vi "addImageToQueue.vi"(8 "error in (no error)":errorcluster, 10 "ImageData":T1, 11 "Camera in":refnum<class "Camera.lvclass">) -> (0 "error out":errorcluster, 3 "Camera out":refnum<class "Camera.lvclass">)   [LabVIEW 2009, in "Hardware.lvlib" / "Channels.lvlib" / "Camera.lvclass"]
uses:
  Camera.lvclass
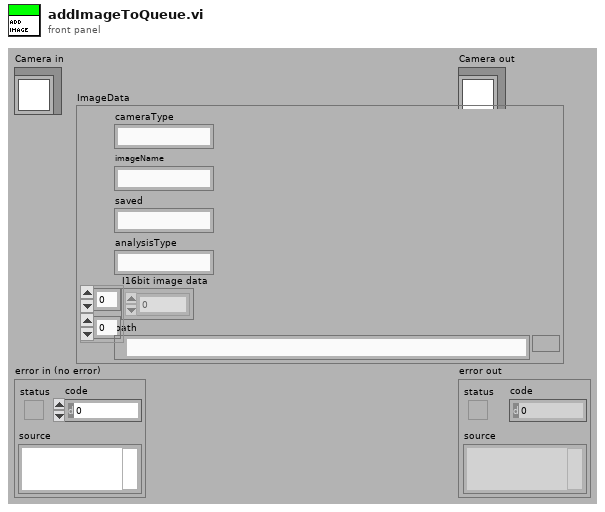
[diagram p1: front panel]
types:
  T1 = cluster{"cameraType":string, "imageName":string, "saved":string, "analysisType":string, "I16bit image data":u16[][], "path":path}
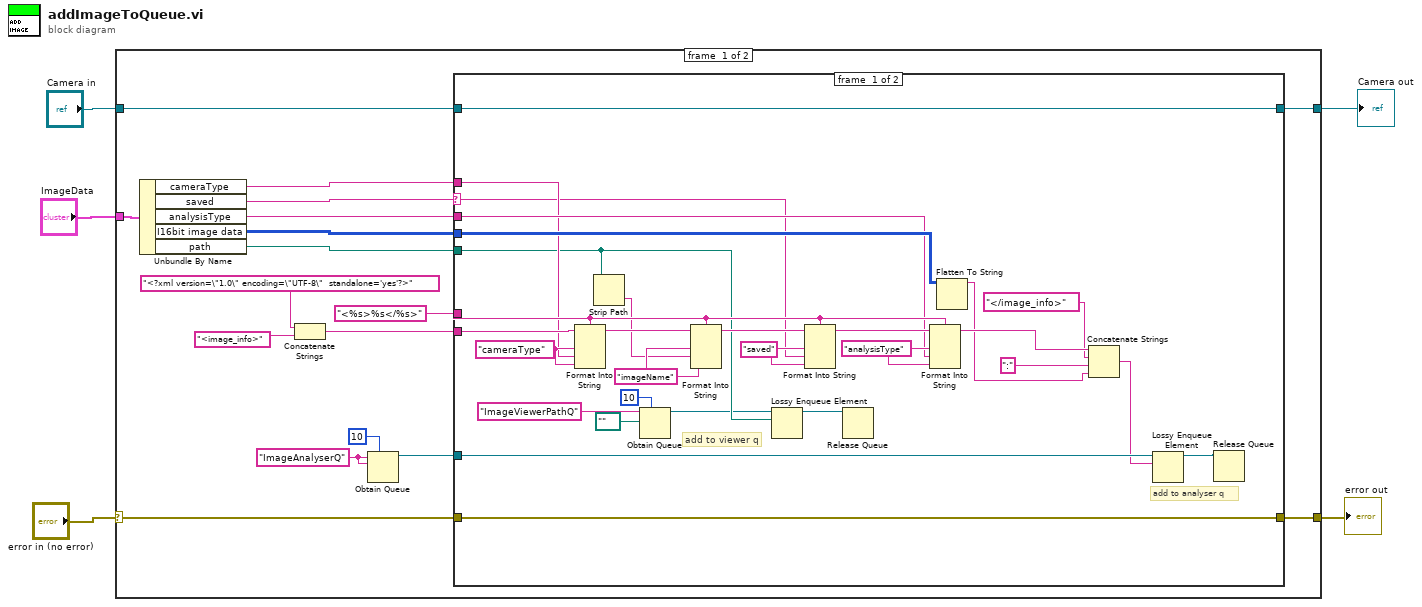
[diagram p0: block diagram]
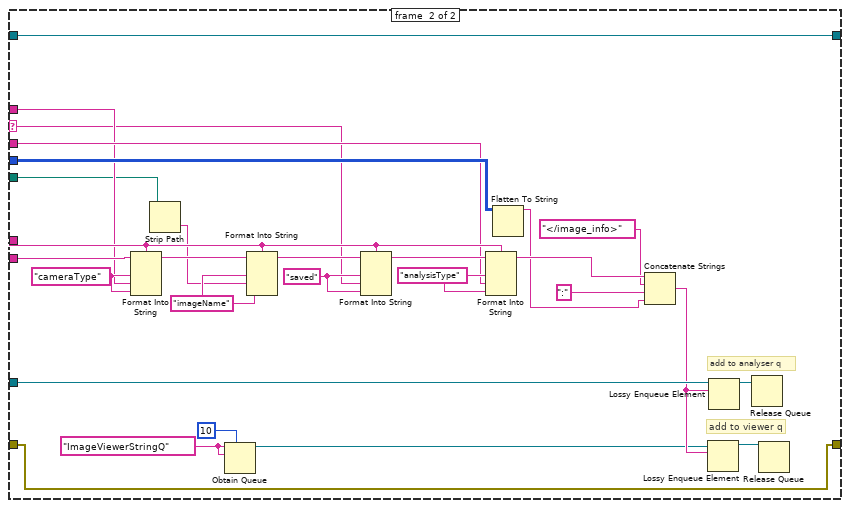
[diagram p2: hidden frame]
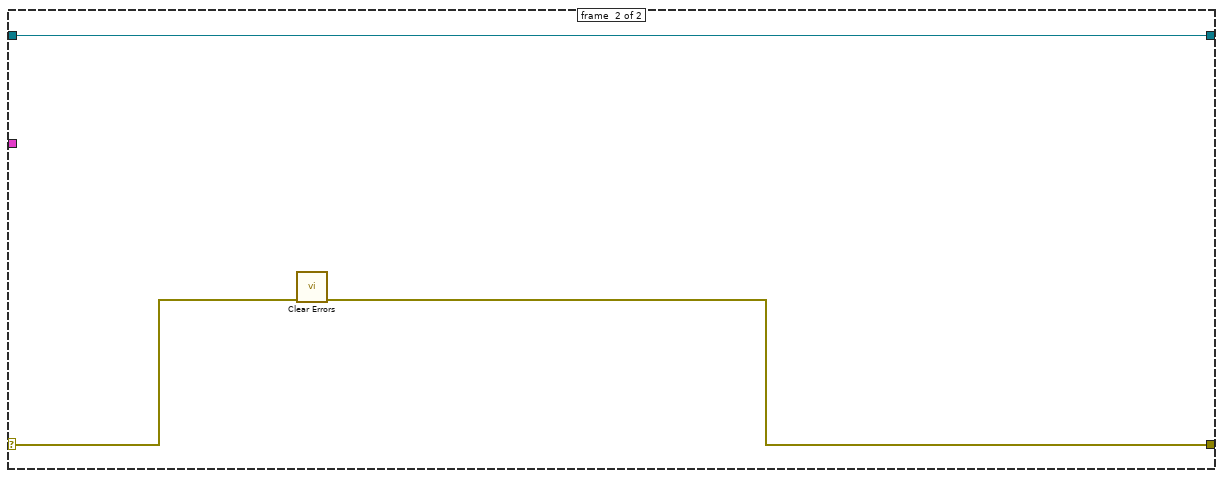
[diagram p3: hidden frame]
diagram:
  n1 = case shown="No Error" "error in (no error)" {
    selector: "error in (no error)" -> [w7 w82]
    tunnel: [w6 w80] -> w4
    tunnel: [w19 w81] -> w2
    tunnel: "Camera in" -> [w21 w81]
    tunnel: "ImageData" -> [w22 _]
    frame #0 {
      w10 = "ImageAnalyserQ"
      n2 = Unbundle By Name(w22) -> ("cameraType"=w18:string, "saved"=w20:string, "analysisType"=w17:string, "I16bit image data"=w16:u16[][], "path"=w15:path)
      n3 = Concatenate Strings("<?xml version=\"1.0\" encoding=\"UTF-8\"  standalone='yes'?>", "<image_info>") -> (w12:string)
      n4 = Obtain Queue(max queue size (-1, unlimited)=10, name (unnamed)=w10, element data type=w10) -> (queue out=w8:refnum<queue>)  [unwired: 2 in, 2 out]
      n5 = case shown="\"true\"" w20 {
        selector: w20 -> [w33 w61]
        tunnel: w21 -> [w51 w79]
        tunnel: [w51 w79] -> w19
        tunnel: w18 -> [w34 w62]
        tunnel: w17 -> [w35 w63]
        tunnel: w16 -> [w37 w65]
        tunnel: w15 -> [w32 w60]
        tunnel: w12 -> [w40 w68]
        tunnel: "<%s>%s</%s>" -> [w39 w67]
        tunnel: w8 -> [w31 w59]
        tunnel: w7 -> [w23 w52]
        tunnel: [w23 w52] -> w6
        frame #0 {
          w48 = "analysisType"
          w46 = "saved"
          w42 = "imageName" ("Key")
          w41 = "cameraType"
          # "add to analyser q"
          # "add to viewer q"
          n6 = Format Into String(format string=w39, initial string=w40, w41, w34, w41) -> (resulting string=w44:string)  [unwired: 1 in, 1 out]
          n7 = Strip Path(path=w32) -> (name=w38:string)  [unwired: 1 out]
          n8 = Obtain Queue(max queue size (-1, unlimited)=10, name (unnamed)="ImageViewerPathQ", element data type=path "") -> (queue out=w26:refnum<queue>)  [unwired: 2 in, 2 out]
          n9 = Format Into String(format string=w39, initial string=w44, w42, w38, w42) -> (resulting string=w45:string)  [unwired: 1 in, 1 out]
          n10 = Lossy Enqueue Element(queue=w26, element=w32) -> (queue out=w25:refnum<queue>)  [unwired: 1 in, 3 out]
          n11 = Format Into String(format string=w39, initial string=w45, w46, w33, w46) -> (resulting string=w49:string)  [unwired: 1 in, 1 out]
          n12 = Release Queue(queue=w25) -> ()  [unwired: 2 in, 3 out]
          n13 = Format Into String(format string=w39, initial string=w49, w48, w35, w48) -> (resulting string=w50:string)  [unwired: 1 in, 1 out]
          n14 = Flatten To String(anything=w37) -> (data string=w36:string)  [unwired: 3 in, 2 out]
          n15 = Concatenate Strings(w50, "</image_info>", ":", w36) -> (w30:string)
          n16 = Lossy Enqueue Element(queue=w31, element=w30) -> (queue out=w24:refnum<queue>)  [unwired: 1 in, 3 out]
          n17 = Release Queue(queue=w24) -> ()  [unwired: 2 in, 3 out]
        }
        frame #1 {
          w56 = "ImageViewerStringQ"
          w76 = "analysisType"
          w74 = "saved"
          w70 = "imageName" ("Key")
          w69 = "cameraType"
          # "add to analyser q"
          # "add to viewer q"
          n18 = Format Into String(format string=w67, initial string=w68, w69, w62, w69) -> (resulting string=w72:string)  [unwired: 1 in, 1 out]
          n19 = Strip Path(path=w60) -> (name=w66:string)  [unwired: 1 out]
          n20 = Obtain Queue(max queue size (-1, unlimited)=10, name (unnamed)=w56, element data type=w56) -> (queue out=w55:refnum<queue>)  [unwired: 2 in, 2 out]
          n21 = Format Into String(format string=w67, initial string=w72, w70, w66, w70) -> (resulting string=w73:string)  [unwired: 1 in, 1 out]
          n22 = Format Into String(format string=w67, initial string=w73, w74, w61, w74) -> (resulting string=w77:string)  [unwired: 1 in, 1 out]
          n23 = Format Into String(format string=w67, initial string=w77, w76, w63, w76) -> (resulting string=w78:string)  [unwired: 1 in, 1 out]
          n24 = Flatten To String(anything=w65) -> (data string=w64:string)  [unwired: 3 in, 2 out]
          n25 = Concatenate Strings(w78, "</image_info>", ":", w64) -> (w58:string)
          n26 = Lossy Enqueue Element(queue=w55, element=w58) -> (queue out=w53:refnum<queue>)  [unwired: 1 in, 3 out]
          n27 = Lossy Enqueue Element(queue=w59, element=w58) -> (queue out=w54:refnum<queue>)  [unwired: 1 in, 3 out]
          n28 = Release Queue(queue=w54) -> ()  [unwired: 2 in, 3 out]
          n29 = Release Queue(queue=w53) -> ()  [unwired: 2 in, 3 out]
        }
      }
    }
    frame #1 {
      n30 = call <vilib>:"Clear Errors.vi"("error in (no error)"=w82) -> ("error out"=w80:errorcluster)  [unwired: 6 in]
    }
  }
  "error out" <- w4
  "Camera out" <- w2
